vi "setPowerLim.vi"(1 "ctlref":T1, 2 "Variant":variant) -> (0 "notification":string)   [LabVIEW 2017]
uses:
  RefArray/RefArray.ctl
panel:
  in  "Cluster":cluster{"abbr":string, "min":dbl, " max":dbl}
  # "Can handle:\n - Matisse power knob\n - Millennia power knob"
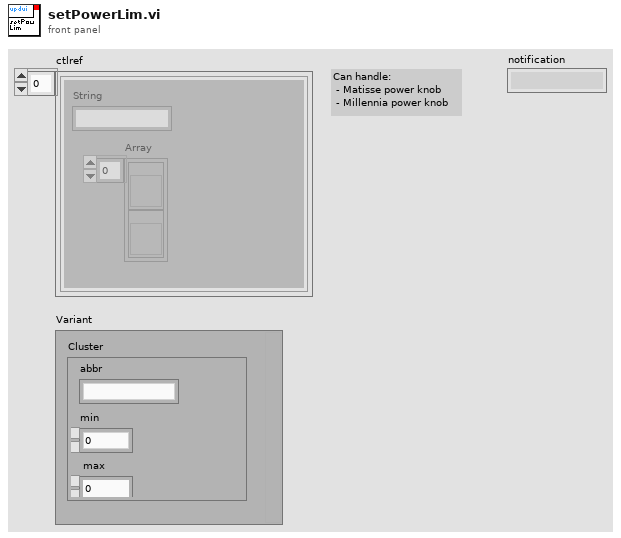
[diagram p1: front panel]
types:
  T1 = typedef "RefArray.ctl" = cluster{"String":string, "Array":refnum<vi>[]}[]
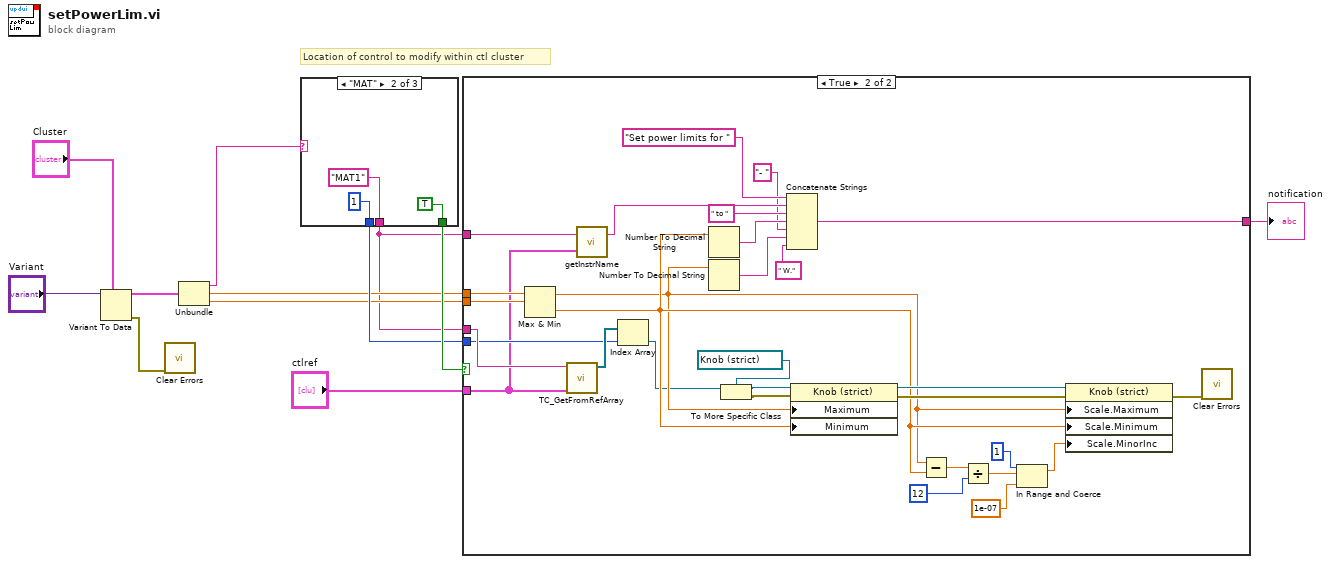
[diagram p0: block diagram]
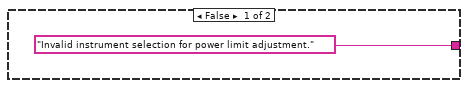
[diagram p2: hidden frame]
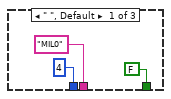
[diagram p3: hidden frame]
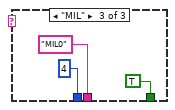
[diagram p4: hidden frame]
diagram:
  # "Location of control to modify within ctl cluster"
  n1 = Variant To Data(type="Cluster", Variant="Variant") -> (data=w8:cluster{"abbr":string, "min":dbl, " max":dbl}, error out=w1:errorcluster)  [unwired: 1 in]
  n2 = call <vilib>:"Clear Errors.vi"("error in (no error)"=w1) -> ()  [unwired: 5 in, 2 out]
  n3 = Unbundle(w8) -> ("abbr"=w7:string, "min"=w6:dbl, "max"=w5:dbl)
  n4 = case shown="\"MAT\"" w7 {
    tunnel: [FALSE TRUE TRUE] -> w11
    tunnel: [4 1 4] -> w10
    tunnel: ["MIL0" "MAT1" "MIL0"] -> w4
    frame " ", Default {
    }
    frame "MAT" {
    }
    frame "MIL" {
    }
  }
  n5 = case shown="True" w11 {
    tunnel: "ctlref" -> [_ w39]
    tunnel: w10 -> [_ w50]
    tunnel: w4 -> [_ w52]
    tunnel: w6 -> [_ w49]
    tunnel: w5 -> [_ w48]
    tunnel: w4 -> [_ w38]
    tunnel: ["Invalid instrument selection for power limit adjustment." w28] -> w3
    frame False {
    }
    frame True {
      n6 = Max & Min(x=w49, y=w48) -> (max(x,y)=w32:dbl, min(x,y)=w35:dbl)
      n7 = call "TC_GetFromRefArray.vi"("arrayIn"=w39, "NameToFind"=w52) -> ("refArray"=w51:refnum<vi>[])  [unwired: 8 in, 1 out]
      n8 = call "getInstrName.vi"("ctlref"=w39, "abbr?"=w38) -> ("name"=w36:string)  [unwired: 1 out]
      n9 = Index Array(array=w51, index=w50) -> (element=w24:refnum<vi>)
      n10 = Number To Decimal String(number=w35) -> (decimal integer string=w33:string)  [unwired: 1 in]
      n11 = Number To Decimal String(number=w32) -> (decimal integer string=w30:string)  [unwired: 1 in]
      n12 = To More Specific Class(target class=refnum<vi> refnum ("reference"), reference=w24) -> (specific class reference=w27:refnum<vi>, error out=w26:errorcluster)  [unwired: 1 in]
      n13 = Concatenate Strings("Set power limits for ", w36, " to ", w33, "- ", w30, " W.") -> (w28:string)
      n14 = property on="Property Node" class="Knob (strict)"(reference=w27, error in=w26, "Maximum"=w32, "Minimum"=w35) -> (reference out=w46:refnum<vi>, error out=w47:errorcluster)
      n15 = Subtract(x=w32, y=w35) -> (x-y=w45:dbl)
      n16 = Divide(x=w45, y=12) -> (x/y=w43:dbl)
      n17 = In Range and Coerce(upper limit=1, x=w43, lower limit=1e-07) -> (coerced(x)=w40:dbl)  [unwired: 1 out]
      n18 = property class="Knob (strict)"(reference=w46, error in=w47, "Scale.Maximum"=w32, "Scale.Minimum"=w35, "Scale.MinorInc"=w40) -> (error out=w23:errorcluster)  [unwired: 1 out]
      n19 = call <vilib>:"Clear Errors.vi"("error in (no error)"=w23) -> ()  [unwired: 5 in, 2 out]
    }
  }
  "notification" <- w3
